vi "create module list.vi"(10 "Instance Identifier":string[](array[string]), 11 "Display Names":string[](array[string])) -> (3 "listbox names":string[](array[string]))   [LabVIEW 2013, in "Standard Engine Editor Node.lvclass"]
uses:
  Standard Engine Editor Node.lvclass
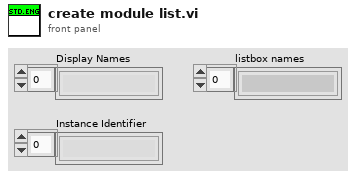
[diagram p1: front panel]
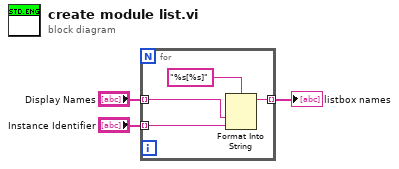
[diagram p0: block diagram]
diagram:
  n1 = for {
    tunnel: "Display Names" -> [w7] mode=indexing
    tunnel: "Instance Identifier" -> [w6] mode=indexing
    tunnel: [w5] -> w3 mode=indexing
    n2 = Format Into String(format string="%s[%s]", w7, w6) -> (resulting string=w5:string)  [unwired: 2 in, 1 out]
  }
  "listbox names" <- w3
